vi "Frame3.vi"   [LabVIEW 2014]
uses:
  QwaveSys_Interface/QwaveSys_Interface.lvlib
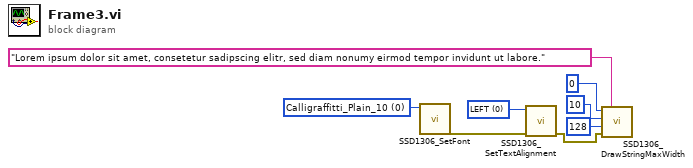
[diagram p0: block diagram]
diagram:
  w1 = u16 0 items=["Calligraffitti_Plain_10", "ArialMT_Plain_10", "ArialMT_Plain_16", "ArialMT_Plain_24"] ("Font")
  w3 = u16 0 items=["LEFT", "CENTER", "RIGHT"] ("alignment")
  n1 = call "SSD1306_SetFont.vi"("Font"=w1) -> ("error out"=w2:errorcluster)  [unwired: 10 in]
  n2 = call "SSD1306_SetTextAlignment.vi"("error in (no error)"=w2, "alignment"=w3) -> ("error out"=w4:errorcluster)  [unwired: 9 in]
  n3 = call "SSD1306_DrawStringMaxWidth.vi"("String"="Lorem ipsum dolor sit amet, consetetur sadipscing elitr, sed diam nonumy eirmod tempor invidunt ut labore.", "error in (no error)"=w4, "max line width"=u8 128, "y"=u8 10, "x"=u8 0) -> ()  [unwired: 6 in, 1 out]
